vi "create.exclude_task.vi"(10 "topic":string[](array[string])) -> (3 "Exclude Filter":refnum<class "exclude.lvclass">)   [LabVIEW 2020, in "nominal types.lvlib" / "channelFilter.lvlib" / "channelFilter.lvclass"]
uses:
  channelFilter.lvclass
  exclude/exclude.lvclass
  topic/topic.lvclass
  C:/code/labview-client/lv_src/nominal types/filterTypes/filterTypes.lvclass
  topic/topic.lvclass/topic.ctl
  exclude/exclude.lvclass/exclude.ctl
  topic/topic.set.vi
  exclude/exclude.set.vi
  filterTypes/filterTypes.lvclass
  channelFilter.lvclass/channelFilter.ctl
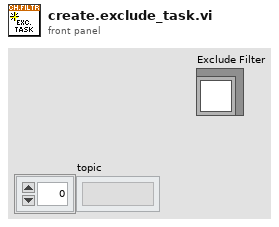
[diagram p1: front panel]
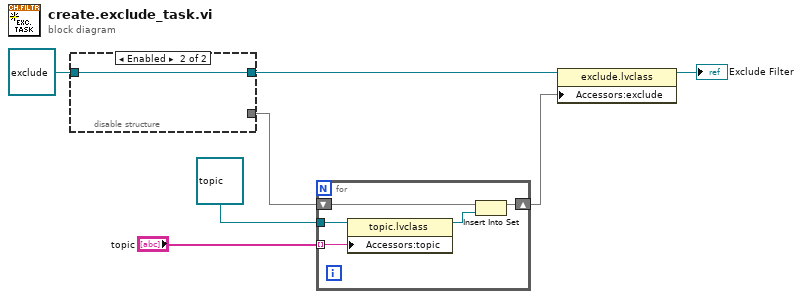
[diagram p0: block diagram]
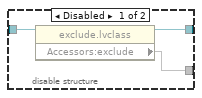
[diagram p2: hidden frame]
diagram:
  n1 = disable-structure shown="Enabled" {
    disable-tunnel: refnum<class "exclude.lvclass"> refnum ("Exclude Filter") -> [w10 w11]
    disable-tunnel: [w9 w11] -> w4
    disable-tunnel: [w8 _] -> w3
    frame Disabled {
      n2 = property class="exclude.lvclass"(reference=w10) -> (reference out=w9:refnum<class "exclude.lvclass">, "Accessors:exclude"=w8:set{refnum<class "filterTypes.lvclass">})  [unwired: 1 in, 1 out]
    }
    frame Enabled {
    }
  }
  n3 = for {
    tunnel: refnum<class "topic.lvclass"> refnum ("nominal types.lvlib:channelFilter.lvlib:topic.lvclass") -> [w16]
    shift-right: [w13] -> w7
    shift-left: w3 -> [w15]
    tunnel: "topic" -> [w12] mode=indexing
    n4 = property class="topic.lvclass"(reference=w16, "Accessors:topic"=w12) -> (reference out=w14:refnum<class "topic.lvclass">)  [unwired: 1 in, 1 out]
    n5 = Insert Into Set(10:w14, 11:w15) -> (3:w13:set{refnum<class "filterTypes.lvclass">})  [unwired: 1 out]
  }
  n6 = property class="exclude.lvclass"(reference=w4, "Accessors:exclude"=w7) -> (reference out=→"Exclude Filter":refnum<class "exclude.lvclass">)  [unwired: 1 in, 1 out]
